vi "Single Tone Measurement (IO).vi"(7 "stop generation":bool=TRUE, 8 "error in (no error)":errorcluster, 11 "measurement configuration":T4={"digital channel list"="", "frame clock rate"=0.0, "number of channels"=0, "channel length"=0, "bit depth"=0, "data justification"=enum."Left Justified", "endianness"=enum."MSB First", "bit clock edge sync"=enum."Rising", "frame sync edge for channel 0"=enum."Rising", "channel 0 offset"=0, "master clock channel list"="", "master clock rate"=0.0, "enable dither"=FALSE, "logic level"=enum."3.3 V", "signal frequency"=1000.0, "output level"=0.0, "output level units"=enum."% FS", "output range (pk-pk)"=0.0, "load impedance"=0.0, "signal phase"=0.0, "acq sampling rate"=0.0, "min measurement cycles"=0, "min measurement time (s)"=0.0, "min settling cycles"=0, "min settling time (s)"=0.0, "acq channel"="", "band start"=0.0, "band stop"=0.0, "weighting filter"=enum."Linear", "highpass filter"=enum."DC", "lowpass filter"=enum."No filter", "SNR units"=enum."dB", "THD+N units"=enum."dB", "THD units"=enum."dB", "gain units"=enum."dB"} {"signal phase" format="%0.2f"; "master clock rate" format="%#_6pHz"; "frame clock rate" format="%#_6pHz"}) -> (0 "error out":errorcluster, 1 "spectra":cluster{"x0":dbl, "dx":dbl, "magnitude":dbl[]}[](array[cluster]), 2 "waveforms":waveform(dbl)[](array[waveform]), 3 "results":T1[](array[typedef]), 4 "output power":dbl[](array[numeric]), 5 "PCM tasks":T2)   [LabVIEW 2021]
uses:
  controls/single tone measurement settings (HW).ctl
  controls/digital audio protocol/data justification.ctl
  controls/digital audio protocol/endianness.ctl
  controls/digital audio protocol/digital edge.ctl
  controls/digital audio protocol/logic level.ctl
  controls/digital output level units.ctl
  controls/weighting filter.ctl
  controls/highpass filter.ctl
  controls/lowpass filter.ctl
  controls/units - snr.ctl
  controls/units - ratio.ctl
  controls/digital audio protocol/PCM tasks.ctl
  <vilib>/PDM Acquisition Toolkit/host/Classes/Tasks/PCM Output/Controls/PCM Output Task DVR.ctl
  <vilib>/PDM Acquisition Toolkit/host/Classes/Tasks/PCM Output/PCM Output Task.lvclass
  <vilib>/PDM Acquisition Toolkit/shared/controls/clock mode.ctl
  <vilib>/PDM Acquisition Toolkit/shared/controls/PCM Frame Sync Control.ctl
  <vilib>/PDM Acquisition Toolkit/shared/controls/Digital Edge.ctl
  <vilib>/PDM Acquisition Toolkit/shared/controls/PCM Data Format Configuration.ctl
  <vilib>/PDM Acquisition Toolkit/shared/controls/PCM Bit Endianness.ctl
  <vilib>/PDM Acquisition Toolkit/shared/controls/PCM Data Justification.ctl
  controls/single tone audio measurement settings.ctl
  controls/audio filter settings.ctl
  controls/units settings.ctl
  <vilib>/DAQmx/read.llb/DAQmx Read (Analog 1D Wfm NChan NSamp).vi
  <vilib>/DAQmx/create/channels.llb/DAQmx Create Channel (AI-Voltage-Basic).vi
  <vilib>/DAQmx/configure/timing.llb/DAQmx Timing (Sample Clock).vi
  <vilib>/PDM Acquisition Toolkit/host/API/Public/Function Generator/Configure Custom Signal (N Ch) - PCM Output Task.vi
  <vilib>/DAQmx/miscellaneous.llb/DAQmx Fill In Error Info.vi
  <vilib>/Waveform/WDTOps.llb/WDT Get Waveform Subset DBL.vi
  <vilib>/PDM Acquisition Toolkit/shared/PDM Shared.lvlib
  <vilib>/PDM Acquisition Toolkit/host/API/PDM Acquisition Toolkit.lvlib
  controls/audio controls.lvlib
  controls/single tone audio measurements.ctl
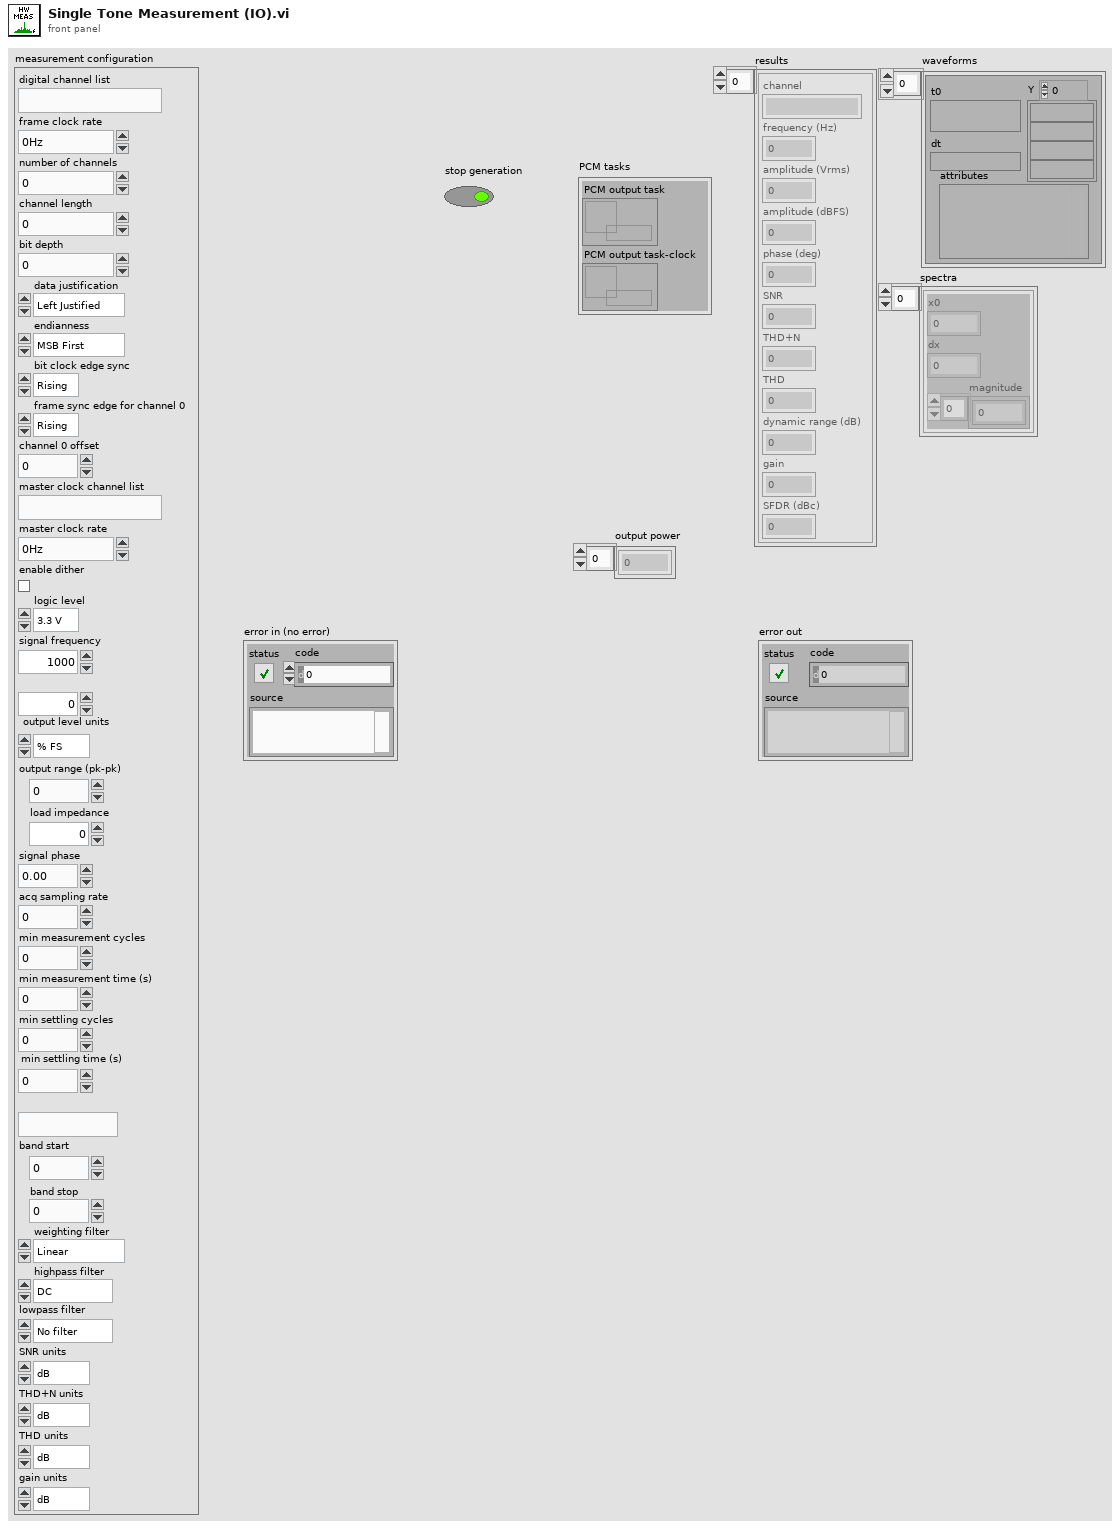
[diagram p1: front panel]
types:
  T1 = typedef "audio controls.lvlib/single tone audio measurements.ctl" = cluster{"channel":string, "frequency (Hz)":dbl, "amplitude (Vrms)":dbl, "amplitude (dBFS)":dbl, "phase (deg)":dbl, "SNR":dbl, "THD+N":dbl, "THD":dbl, "dynamic range (dB)":dbl, "gain":dbl, "SFDR (dBc)":dbl}
  T2 = typedef "PCM tasks.ctl" = cluster{"PCM output task":T3, "PCM output task-clock":T3}
  T3 = typedef "PDM Acquisition Class Library.lvlib/PCM Output Task.lvclass/PCM Output Task DVR.ctl" = refnum<data-value>
  T4 = typedef "single tone measurement settings (HW).ctl" = cluster{"digital channel list":string, "frame clock rate":dbl, "number of channels":u32, "channel length":u32, "bit depth":u32, "data justification":T5, "endianness":T6, "bit clock edge sync":T7, "frame sync edge for channel 0":T7, "channel 0 offset":u32, "master clock channel list":string, "master clock rate":dbl, "enable dither":bool, "logic level":T8, "signal frequency":dbl, "output level":dbl, "output level units":T9, "output range (pk-pk)":dbl, "load impedance":dbl, "signal phase":dbl, "acq sampling rate":dbl, "min measurement cycles":u32, "min measurement time (s)":dbl, "min settling cycles":u32, "min settling time (s)":dbl, "acq channel":string, "band start":dbl, "band stop":dbl, "weighting filter":T10, "highpass filter":T11, "lowpass filter":T12, "SNR units":T13, "THD+N units":T14, "THD units":T14, "gain units":T14}
  T5 = typedef "data justification.ctl" = enum32{"Left Justified", "Right Justified"}
  T6 = typedef "endianness.ctl" = enum32{"MSB First", "LSB First"}
  T7 = typedef "digital edge.ctl" = enum32{"Rising", "Falling"}
  T8 = typedef "logic level.ctl" = enum32{"3.3 V", "1.8 V", "1.2 V"}
  T9 = typedef "audio controls.lvlib/digital output level units.ctl" = enum32{"% FS", "dBFS"}
  T10 = typedef "weighting filter.ctl" = enum32{"Linear", "A-weighting", "B-weighting", "C-weighting"}
  T11 = typedef "highpass filter.ctl" = enum32{"DC", "AC"}
  T12 = typedef "lowpass filter.ctl" = enum32{"No filter", "AES17 20kHz", "AES17 40kHz"}
  T13 = typedef "audio controls.lvlib/units - snr.ctl" = enum32{"dB", "x/y"}
  T14 = typedef "audio controls.lvlib/units - ratio.ctl" = enum32{"dB", "%", "x/y"}
  T15 = typedef "audio controls.lvlib/units settings.ctl" = cluster{"SNR units":T13, "THD+N units":T14, "THD units":T14, "gain units":T14}
  T16 = typedef "audio filter settings.ctl" = cluster{"weighting filter":T10, "highpass filter":T11, "lowpass filter ":T12}
  T17 = typedef "single tone audio measurement settings.ctl" = cluster{"Band start":dbl, "Band stop":dbl, "Amplitude":dbl, "Frequency":dbl, "Full scale range":dbl}
  T18 = typedef "PDM Shared.lvlib/PCM Data Format Configuration.ctl" = cluster{"Frame Sync Edge for Channel 0":T19, "Channel Count Per Frame":u8, "Channel Length":u16, "Bit Depth":u8, "Channel 0 Offset":u16, "Endianness":T20, "Data Justification":T21}
  T19 = typedef "PDM Shared.lvlib/Digital Edge.ctl" = enum8{"Rising", "Falling"}
  T20 = typedef "PDM Shared.lvlib/PCM Bit Endianness.ctl" = enum16{"MSB First", "LSB First"}
  T21 = typedef "PDM Shared.lvlib/PCM Data Justification.ctl" = enum16{"Left Justified", "Right Justified"}
  T22 = typedef "PDM Shared.lvlib/PCM Frame Sync Control.ctl" = cluster{"Frame Length":u16, "Frame Sync Pulse Width":u16, "Bit Clock Edge  Sync":T19}
  T23 = typedef "PDM Shared.lvlib/clock mode.ctl" = enum16{"divided clock", "DDS"}
  T24 = typedef "PDM Acquisition Class Library.lvlib/I2S Output Task.lvclass/SignalProperties.ctl" = cluster{"cyclic signal":dbl[], "channel parameters":T25[]}
  T25 = typedef "PDM Acquisition Class Library.lvlib/I2S Output Channel.lvclass/GenerationChannelProperties.ctl" = cluster{"cyclic period":dbl, "cyclic phase offset":dbl, "gain":dbl}
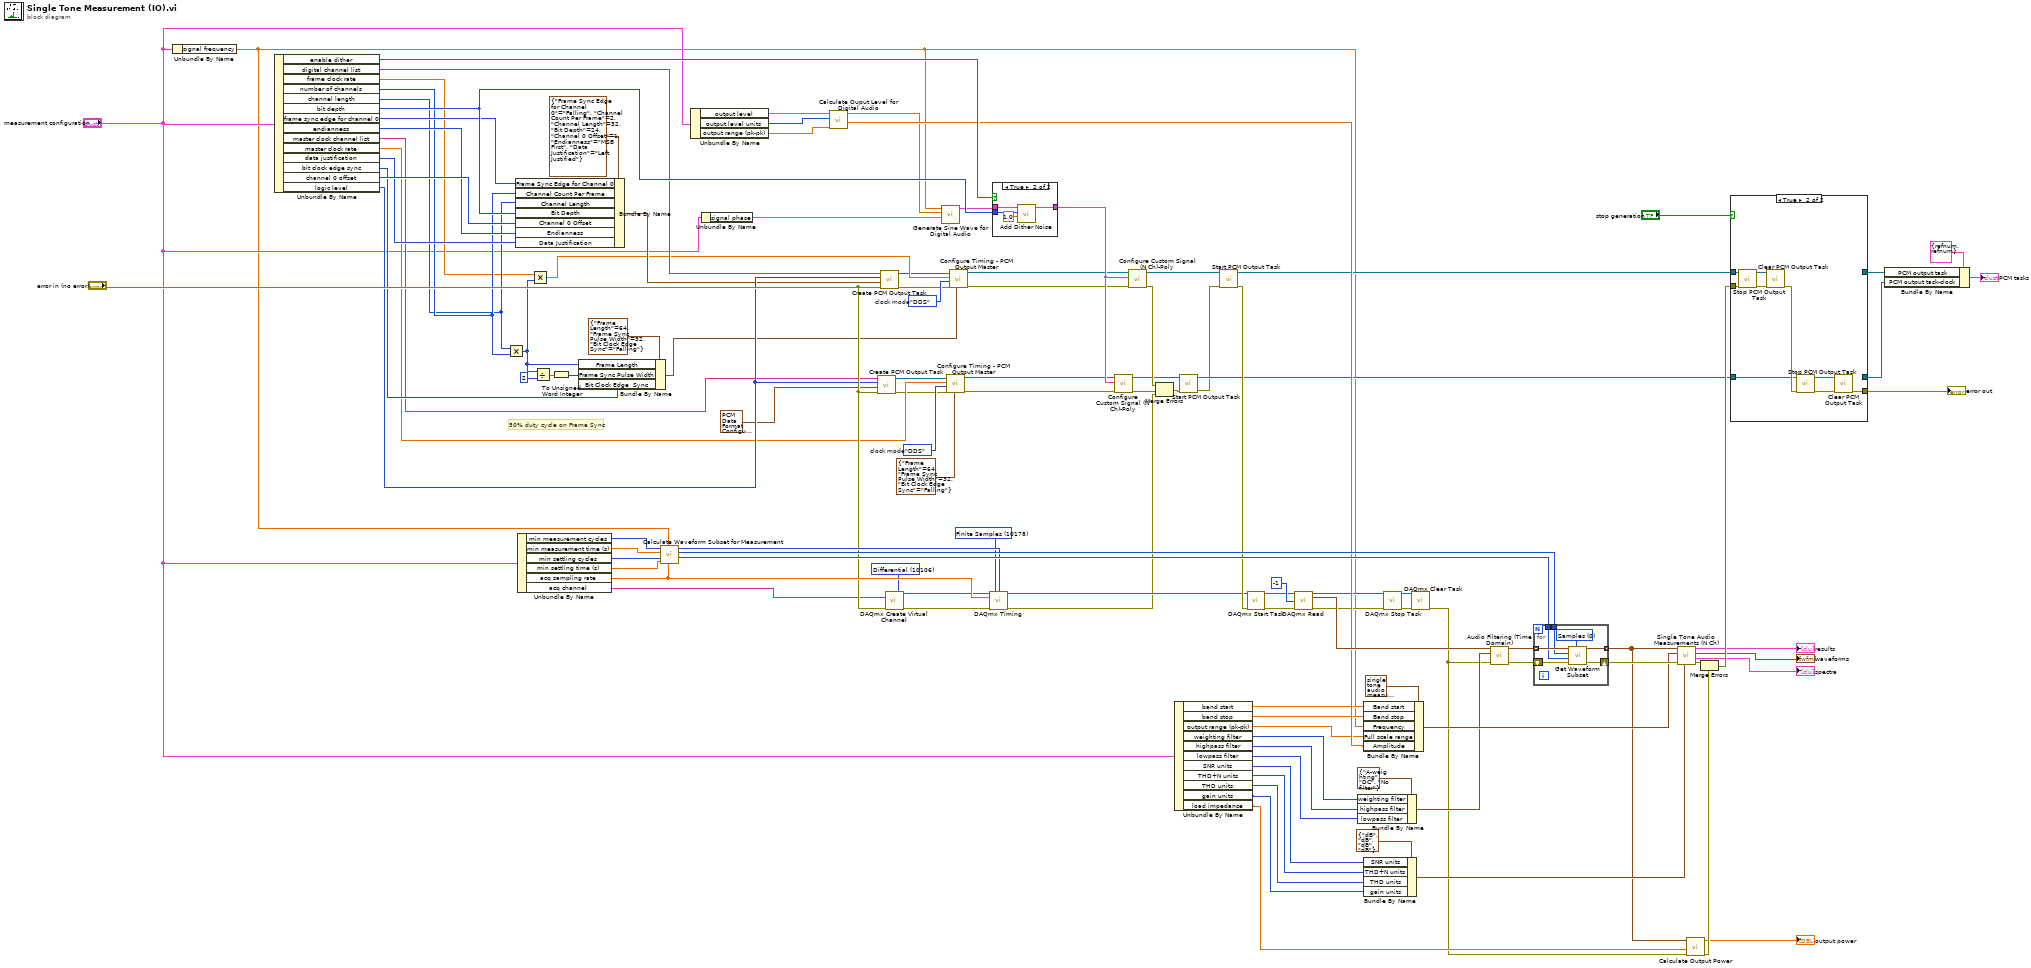
[diagram p0: block diagram]
diagram:
  w61 = 10106 items=["Default"=-1, "RSE"=10083, "NRSE"=10078, "Differential"=10106, "Pseudodifferential"=12529] ("input terminal configuration")
  w50 = 10178 items=["Finite Samples"=10178, "Continuous Samples"=10123, "Hardware Timed Single Point"=12522] ("sample mode")
  w18 = clock_mode."DDS"  # clock mode
  w15 = clock_mode."DDS"  # clock mode
  # "50% duty cycle on Frame Sync"
  n1 = Unbundle By Name("measurement configuration") -> ("signal frequency"=w11:dbl)
  n2 = Unbundle By Name("measurement configuration") -> ("enable dither"=w113:bool, "digital channel list"=w74:string, "frame clock rate"=w52:dbl, "number of channels"=w54:u32, "channel length"=w53:u32, "bit depth"=w112:u32, "frame sync edge for channel 0"=w64:T7, "endianness"=w65:T6, "master clock channel list"=w55:string, "master clock rate"=w56:dbl, "data justification"=w63:T5, "bit clock edge sync"=w66:T7, "channel 0 offset"=w67:u32, "logic level"=w68:T8)
  n3 = Multiply(x=w53, y=w54) -> (x*y=w29:u32)
  n4 = Bundle By Name(cluster=T18 {"Frame Sync Edge for Channel 0"=enum."Falling", "Channel Count Per Frame"=2, "Channel Length"=32, "Bit Depth"=24, "Channel 0 Offset"=1, "Endianness"=enum."MSB First", "Data Justification"=enum."Left Justified"} ("PCM Data Configuration"), "Frame Sync Edge for Channel 0"=w64, "Channel Count Per Frame"=w54, "Channel Length"=w53, "Bit Depth"=w112, "Channel 0 Offset"=w67, "Endianness"=w65, "Data Justification"=w63) -> (w32:T18)
  n5 = Unbundle By Name("measurement configuration") -> ("min measurement cycles"=w99:u32, "min measurement time (s)"=w100:dbl, "min settling cycles"=w101:u32, "min settling time (s)"=w102:dbl, "acq sampling rate"=w91:dbl, "acq channel"=w60:string)
  n6 = Multiply(x=w52, y=w29) -> (x*y=w30:dbl)
  n7 = Divide(x=w29, y=u16 2) -> (x/y=w27:dbl)
  n8 = To Unsigned Word Integer(number=w27) -> (unsigned 16bit integer=w28:u16)
  n9 = Bundle By Name(cluster=T22 {"Frame Length"=64, "Frame Sync Pulse Width"=32, "Bit Clock Edge  Sync"=enum."Falling"} ("Frame Sync Clock Control"), "Frame Length"=w29, "Frame Sync Pulse Width"=w28, "Bit Clock Edge  Sync"=w66) -> (w25:T22)
  n10 = call "Calculate Waveform Subset for Measurement.vi"("sampling rate"=w91, "signal frequency"=w11, "minimum settling duration"=w102, "minimum settling cycles"=w101, "minimum measurement duration"=w100, "minimum measurement cycles"=w99) -> ("duration (samples)"=w98:u32, "start (samples)"=w97:u32, "total acquisition (samples)"=w92:u32)  [unwired: 3 in]
  n11 = Unbundle By Name("measurement configuration") -> ("output level"=w78:dbl, "output level units"=w79:T9, "output range (pk-pk)"=w80:dbl)
  n12 = Unbundle By Name("measurement configuration") -> ("signal phase"=w69:dbl)
  n13 = call "Calculate Ouput Level for Digital Audio.vi"("output range (pk-pk)"=w80, "digital output level units"=w79, "output level"=w78) -> ("amplitude (pk)"=w81:dbl, "gain"=w75:dbl)  [unwired: 7 in]
  n14 = call <vilib>:"Create PCM Output Task.vi"("error in"="error in (no error)", "PCM data configuration"=T18 {"Frame Sync Edge for Channel 0"=enum."Falling", "Channel Count Per Frame"=2, "Channel Length"=32, "Bit Depth"=24, "Channel 0 Offset"=1, "Endianness"=enum."MSB First", "Data Justification"=enum."Left Justified"} ("PCM Data Configuration 2"), "logic level"=w68, "channel list"=w55) -> ("error out"=w17:errorcluster, "PCM output task out"=w16:T3)  [unwired: 6 in]
  n15 = call <vilib>:"Create PCM Output Task.vi"("error in"="error in (no error)", "PCM data configuration"=w32, "logic level"=w68, "channel list"=w74) -> ("error out"=w14:errorcluster, "PCM output task out"=w13:T3)  [unwired: 6 in]
  n16 = call-poly <vilib>:"DAQmx Create Virtual Channel.vi"("input terminal configuration"=w61, "physical channels"=w60, "error in"="error in (no error)") -> ("task out"=w41:refnum<k21>, "error out"=w40:errorcluster)  [unwired: 11 in]
  n17 = call "Generate Sine Wave for Digital Audio.vi"("phase"=w69, "gain"=w75, "frequency"=w11) -> ("Signal Properties"=w110:T24)  [unwired: 8 in]
  n18 = call <vilib>:"Configure Timing - PCM Output Master.vi"("Frame Sync Clock Control"=T22 {"Frame Length"=64, "Frame Sync Pulse Width"=32, "Bit Clock Edge  Sync"=enum."Falling"} ("Frame Sync Clock Control 2"), "error in"=w17, "clock mode"=w18, "Bit Clock rate"=w56, "PCM output task in"=w16) -> ("error out"=w33:errorcluster, "PCM output task out"=w34:T3)  [unwired: 4 in, 1 out]
  n19 = call <vilib>:"Configure Timing - PCM Output Master.vi"("Frame Sync Clock Control"=w25, "error in"=w14, "clock mode"=w15, "Bit Clock rate"=w30, "PCM output task in"=w13) -> ("error out"=w77:errorcluster, "PCM output task out"=w76:T3)  [unwired: 4 in, 1 out]
  n20 = call-poly <vilib>:"DAQmx Timing.vi"("task/channels in"=w41, "sample mode"=w50, "samples per channel"=w92, "rate"=w91, "error in"=w40) -> ("task out"=w49:refnum<k21>, "error out"=w48:errorcluster)  [unwired: 9 in]
  n21 = case shown="True" w113 {
    tunnel: w110 -> [w114 w118]
    tunnel: [w114 w117] -> w111
    tunnel: w112 -> [_ w116]
    frame False {
    }
    frame True {
      n22 = call "Add Dither Noise.vi"("amplitude (LSB)"=1.0, "bits"=w116, "Signal Properties"=w118) -> ("Signal Properties"=w117:T24)  [unwired: 8 in]
    }
  }
  n23 = call-poly <vilib>:"Configure Custom Signal (N Ch)-Poly.vi"("error in"=w33, "signal parameters"=w111, "PCM output task in"=w34) -> ("error out"=w38:errorcluster, "PCM output task out"=w35:T3)  [unwired: 7 in]
  n24 = call-poly <vilib>:"Configure Custom Signal (N Ch)-Poly.vi"("error in"=w77, "signal parameters"=w111, "PCM output task in"=w76) -> ("error out"=w37:errorcluster, "PCM output task out"=w36:T3)  [unwired: 7 in]
  n25 = Merge Errors(w37, w38, w48) -> (w22:errorcluster)
  n26 = Unbundle By Name("measurement configuration") -> ("band start"=w58:dbl, "band stop"=w59:dbl, "output range (pk-pk)"=w73:dbl, "weighting filter"=w88:T10, "highpass filter"=w89:T11, "lowpass filter"=w90:T12, "SNR units"=w105:T13, "THD+N units"=w106:T14, "THD units"=w107:T14, "gain units"=w108:T14, "load impedance"=w109:dbl)
  n27 = call <vilib>:"Start PCM Output Task.vi"("error in"=w22, "PCM output task in"=w35) -> ("error out"=w21:errorcluster, "PCM output task out"=w23:T3)  [unwired: 8 in]
  n28 = call <vilib>:"Start PCM Output Task.vi"("error in"=w21, "PCM output task in"=w36) -> ("error out"=w62:errorcluster, "PCM output task out"=w39:T3)  [unwired: 8 in]
  n29 = call <vilib>:"DAQmx Start Task.vi"("task/channels in"=w49, "error in"=w62) -> ("task out"=w46:refnum<k21>, "error out"=w43:errorcluster)  [unwired: 12 in]
  n30 = call-poly <vilib>:"DAQmx Read.vi"("task/channels in"=w46, "number of samples per channel"=-1, "error in"=w43) -> ("task out"=w47:refnum<k21>, "data"=w93:waveform(dbl)[], "error out"=w44:errorcluster)  [unwired: 10 in]
  n31 = Bundle By Name(cluster=T16 {"weighting filter"=enum."A-weighting", "highpass filter"=enum."DC", "lowpass filter "=enum."No filter"} ("filter settings"), "weighting filter"=w88, "highpass filter"=w89, "lowpass filter"=w90) -> (w86:T16)
  n32 = Bundle By Name(cluster=T17 {"Band start"=20.0, "Band stop"=20000.0, "Amplitude"=-1.0, "Frequency"=1000.0, "Full scale range"=15.0} ("measurement settings"), "Band start"=w58, "Band stop"=w59, "Frequency"=w11, "Full scale range"=w73, "Amplitude"=w81) -> (w87:T17)
  n33 = Bundle By Name(cluster=T15 {"SNR units"=enum."dB", "THD+N units"=enum."dB", "THD units"=enum."dB", "gain units"=enum."dB"} ("units settings"), "SNR units"=w105, "THD+N units"=w106, "THD units"=w107, "gain units"=w108) -> (w104:T15)
  n34 = call <vilib>:"DAQmx Stop Task.vi"("task/channels in"=w47, "error in"=w44) -> ("task out"=w42:refnum<k21>, "error out"=w45:errorcluster)  [unwired: 12 in]
  n35 = call <vilib>:"DAQmx Clear Task.vi"("task in"=w42, "error in"=w45) -> ("error out"=w84:errorcluster)  [unwired: 13 in]
  n36 = call "Audio Filtering (Time Domain).vi"("waveforms"=w93, "filter settings"=w86, "error in"=w84) -> ("time domain"=w95:waveform(dbl)[], "error out"=w94:errorcluster)  [unwired: 6 in]
  n37 = for {
    tunnel: w95 -> [w125] mode=indexing
    tunnel: [w124] -> w5 mode=indexing
    shift-right: [w121] -> w96
    shift-left: w94 -> [w122]
    tunnel: w97 -> [w120]
    tunnel: w98 -> [w119]
    w123 = u16 0 items=["Samples", "Relative Time"] ("start/duration format")
    n38 = call-poly <vilib>:"Get Waveform Subset.vi"("start/duration format"=w123, "error in (no error)"=w122, "duration"=w119, "start samples/time"=w120, "waveform in"=w125) -> ("error out"=w121:errorcluster, "waveform out"=w124:waveform(dbl))  [unwired: 1 in, 2 out]
  }
  n39 = call "Single Tone Audio Measurements (N Ch).vi"("units settings"=w104, "error in"=w96, "measurement settings"=w87, "waveforms"=w5) -> ("error out"=w70:errorcluster, "spectra"=→"spectra":cluster{"x0":dbl, "dx":dbl, "magnitude":dbl[]}[], "waveforms"=→"waveforms":waveform(dbl)[], "results"=→"results":T1[])  [unwired: 4 in]
  n40 = call "Calculate Output Power.vi"("error in (no error)"=w84, "load impedance"=w109, "waveforms"=w5) -> ("error out"=w72:errorcluster, "output power"=→"output power":dbl[])  [unwired: 7 in]
  n41 = Merge Errors(w70, w72) -> (w71:errorcluster)
  n42 = case shown="True" "stop generation" {
    tunnel: [w128 w137] -> w83
    tunnel: w71 -> [w128 w136]
    tunnel: w39 -> [w127 w135]
    tunnel: w23 -> [w126 w133]
    tunnel: [w127 _] -> w9
    tunnel: [w126 _] -> w6
    frame False {
    }
    frame True {
      n43 = call <vilib>:"Stop PCM Output Task.vi"("error in"=w136, "PCM output task In"=w135) -> ("error out"=w129:errorcluster, "PCM output task out"=w130:T3)  [unwired: 8 in]
      n44 = call <vilib>:"Clear PCM Output Task.vi"("error in"=w129, "PCM output task in"=w130) -> ("error out"=w134:errorcluster)  [unwired: 9 in]
      n45 = call <vilib>:"Stop PCM Output Task.vi"("error in"=w134, "PCM output task In"=w133) -> ("error out"=w131:errorcluster, "PCM output task out"=w132:T3)  [unwired: 8 in]
      n46 = call <vilib>:"Clear PCM Output Task.vi"("error in"=w131, "PCM output task in"=w132) -> ("error out"=w137:errorcluster)  [unwired: 9 in]
    }
  }
  "error out" <- w83
  n47 = Bundle By Name(cluster=T2 {"PCM output task"=refnum, "PCM output task-clock"=refnum} ("PCM tasks"), "PCM output task"=w9, "PCM output task-clock"=w6) -> (→"PCM tasks":T2)
